vi "get waveform.vi"(10 "Amplitude":dbl=1.0, 11 "Frequency":dbl=10.1) -> (3 "Array - Numeric":dbl[](array[numeric]))   [LabVIEW 2025]
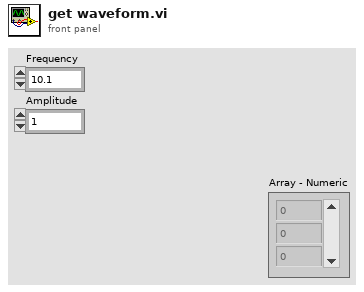
[diagram p1: front panel]
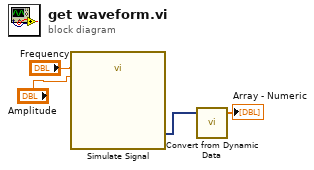
[diagram p0: block diagram]
diagram:
  n1 = call "Simulate Signal"("Frequency"="Frequency", "Amplitude"="Amplitude") -> ("Sine"=w4:dynamicdata)  [unwired: 12 in, 1 out]
  n2 = call "Convert from Dynamic Data"("Dynamic Data Type"=w4) -> ("Array"=→"Array - Numeric":dbl[])  [unwired: 3 in]
